vi "test.vi"() -> ()   [LabVIEW 2020, in "PicoscopeV2.lvclass"]
uses:
  PicoscopeV2.lvclass
panel:
  out "error out":errorcluster
  out "USB 3.0 device on non-USB 3.0 Port":bool
  out "USB Powered":bool=TRUE
  out "Device Info":T1={"Driver Version"="2.1.104.3324", "USB Version"="2.0", "Hardware"="1", "Variant"="5244A", "Batch and Serial"="CQ178/007", "Cal Date"="11Jun13", "Kernel Version"="1.0", "Digital HW Version"="1", "Analogue HW Version"="1", "MSO"=FALSE, "Number of channels"=2}
  in  "Resolution":u32(ring) items=["8-bit"=0, "12-bit"=1, "14-bit"=2, "15-bit"=3, "16-bit"=4, "10-bit"=10]
  in  "Serial Number":string
  in  "Use Serial Number":bool
  in  "error in (no error)":errorcluster
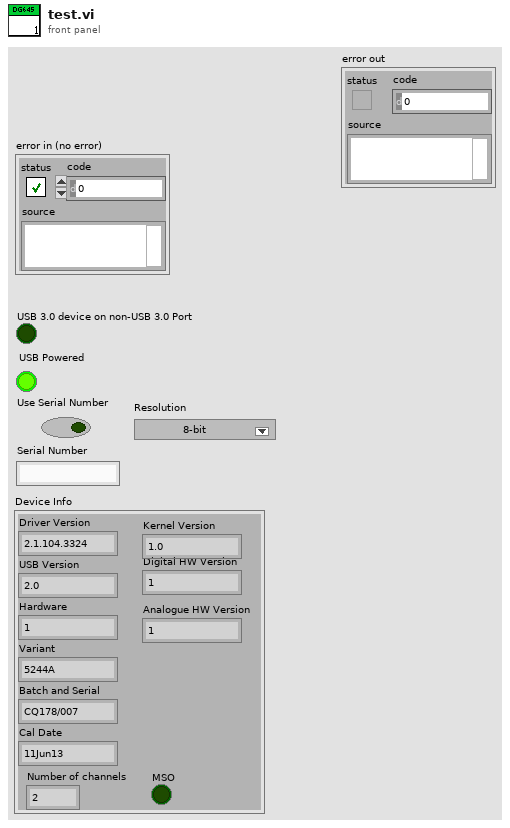
[diagram p1: front panel]
types:
  T1 = cluster{"Driver Version":string, "USB Version":string, "Hardware":string, "Variant":string, "Batch and Serial":string, "Cal Date":string, "Kernel Version":string, "Digital HW Version":string, "Analogue HW Version":string, "MSO":bool, "Number of channels":i16}
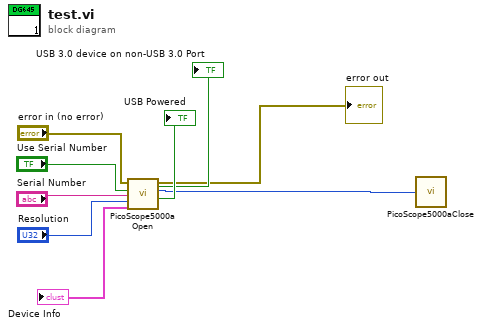
[diagram p0: block diagram]
diagram:
  n1 = call "PicoScope5000aOpen.vi"("Serial Number"="Serial Number", "Resolution"="Resolution", "Use Serial Number"="Use Serial Number", "error in (no error)"="error in (no error)") -> ("USB Powered"=→"USB Powered":bool, "handle"=w2:i16, "error out"=→"error out":errorcluster, "USB 3.0 device on non-USB 3.0 Port"=→"USB 3.0 device on non-USB 3.0 Port":bool, "Device Info"=→"Device Info":T1)  [unwired: 2 in, 1 out]
  n2 = call "PicoScope5000aClose.vi"("handle"=w2) -> ()
